vi "add_code.vi"(1 "add_code":bool, 2 "A":T2) -> (0 "Result":T1)   [LabVIEW 2013]
panel:
  # "R1"
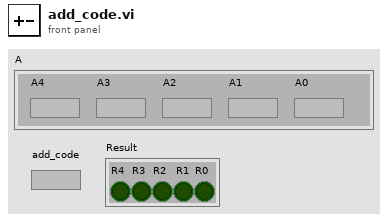
[diagram p1: front panel]
types:
  T1 = cluster{"R4":bool, "R3":bool, "R2":bool, bool, "R0":bool}
  T2 = cluster{"A4":bool, "A3":bool, "A2":bool, "A1":bool, "A0":bool}
  T3 = cluster{"Y5":bool, "Y4":bool, "Y3":bool, "Y2":bool, "Y1":bool, "Y0":bool}
  T4 = cluster{"Y4":bool, "Y3":bool, "Y2":bool, "Y1":bool, "Y0":bool}
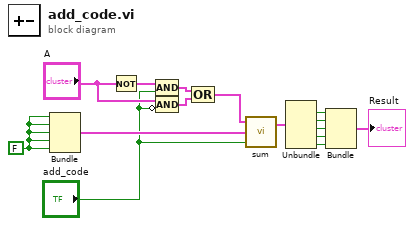
[diagram p0: block diagram]
diagram:
  w15 = FALSE
  n1 = Bundle(w15, w15, w15, w15, w15) -> (w14:cluster{bool, bool, bool, bool, bool})  [unwired: 1 in]
  n2 = Not(x="A") -> (.not. x?=w13:T2)
  n3 = Compound Arithmetic op=AND(w13, "add_code") -> (w10:T2)
  n4 = Compound Arithmetic op=AND("A", invert "add_code") -> (w11:T2)
  n5 = Compound Arithmetic op=OR(w10, w11) -> (w9:T2)
  n6 = call "sum.vi"("+1"="add_code", "B"=w14, "A"=w9) -> ("Output"=w7:T3)  [unwired: 1 out]
  n7 = Unbundle(w7) -> ("Y4"=w6:bool, "Y3"=w5:bool, "Y2"=w4:bool, "Y1"=w3:bool, "Y0"=w2:bool)  [unwired: 1 out]
  n8 = Bundle("Y4"=w6, "Y3"=w5, "Y2"=w4, "Y1"=w3, "Y0"=w2) -> (→"Result":T4)  [unwired: 1 in]
